vi "Perform Action.vi"(8 "error in (no error)":errorcluster, 10 "Input":variant, 11 "object in":refnum<class "Fetch Waveforms CFG.lvclass">) -> (0 "error out":errorcluster, 2 "Output":variant, 3 "object out":refnum<class "Fetch Waveforms CFG.lvclass">)   [LabVIEW 2023, in "Scope Simulated CFGs.lvlib" / "Fetch Waveforms CFG.lvclass"]
uses:
  Fetch Waveforms CFG.lvclass
  Fetch Waveforms CFG.lvclass/Fetch Waveforms CFG.ctl
  <vilib>/ErrorRing/Error Ring.xnode
  <vilib>/Utility/error.llb/Error Cluster From Error Code.vi
  Configuration/Configuration Semaphore/CFG Semaphore.lvclass
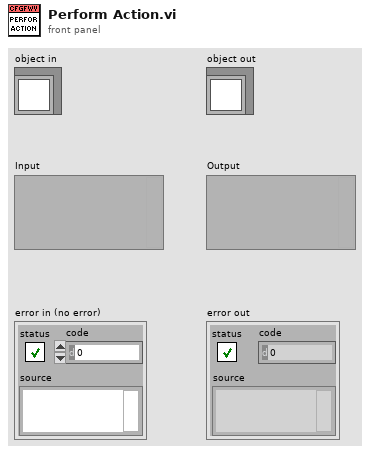
[diagram p1: front panel]
types:
  T1 = typedef "Semaphore RefNum" = refnum<k1>
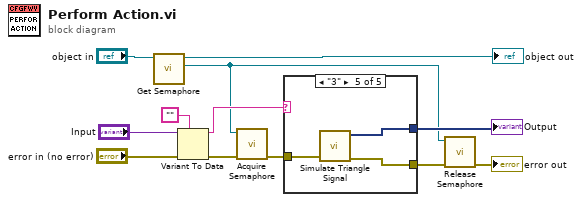
[diagram p0: block diagram]
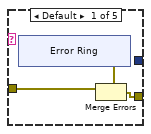
[diagram p2: hidden frame]
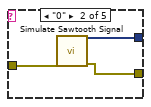
[diagram p3: hidden frame]
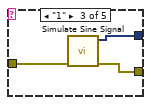
[diagram p4: hidden frame]
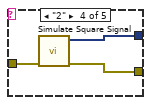
[diagram p5: hidden frame]
diagram:
  n1 = call "Get Semaphore.vi"("CFG Base in"="object in") -> ("Semaphore"=w1:T1, "CFG Base out"=→"object out":refnum<class "Fetch Waveforms CFG.lvclass">)  [unwired: 9 in]
  n2 = Variant To Data(error in="error in (no error)", type="", Variant="Input") -> (data=w9:string, error out=w5:errorcluster)
  n3 = call <vilib>:"Acquire Semaphore.vi"("error in (no error)"=w5, "semaphore"=w1) -> ("error out"=w4:errorcluster)  [unwired: 3 in, 2 out]
  n4 = case shown="\"3\"" w9 {
    tunnel: [_ w23 w26 w28 w30] -> w6
    tunnel: w4 -> [w15 w22 w25 w27 w32]
    tunnel: [w14 w21 w24 w29 w31] -> w7
    frame Default {
      n5 = xnode "Error Ring"() -> ("error out"=w13:errorcluster)
      n6 = Merge Errors(w15, w13) -> (w14:errorcluster)
    }
    frame "0" {
      n7 = call "Simulate Sawtooth Signal.vi"("error in (no error)"=w22) -> ("error out"=w21:errorcluster, "Sawtooth with Uniform Noise"=w23:dynamicdata)  [unwired: 9 in]
    }
    frame "1" {
      n8 = call "Simulate Sine Signal.vi"("error in (no error)"=w25) -> ("error out"=w24:errorcluster, "Sine"=w26:dynamicdata)  [unwired: 9 in]
    }
    frame "2" {
      n9 = call "Simulate Square Signal.vi"("error in"=w27) -> ("error out"=w29:errorcluster, "Square with Uniform Noise"=w28:dynamicdata)  [unwired: 9 in]
    }
    frame "3" {
      n10 = call "Simulate Triangle Signal.vi"("error in (no error)"=w32) -> ("error out"=w31:errorcluster, "Triangle with Uniform Noise"=w30:dynamicdata)  [unwired: 9 in]
    }
  }
  "Output" <- w6
  n11 = call <vilib>:"Release Semaphore.vi"("error in (no error)"=w7, "semaphore"=w1) -> ("error out"=→"error out":errorcluster)  [unwired: 4 in, 1 out]
